vi "RFmx_Cntr_Init_Complete.vi"(7 "Meas_Type":string[](array[string])=["ACP"], 8 "error in (no error)":errorcluster, 11 "Instrument Handle in":refnum<k21>="VST") -> (0 "error out":errorcluster, 3 "Instrument Handle out":refnum<k21>="VST")   [LabVIEW 2014]
uses:
  <vilib>/RFmx/RFInstr/mx/RFmxInstr.llb/RFmxInstr Build Signal String.vi
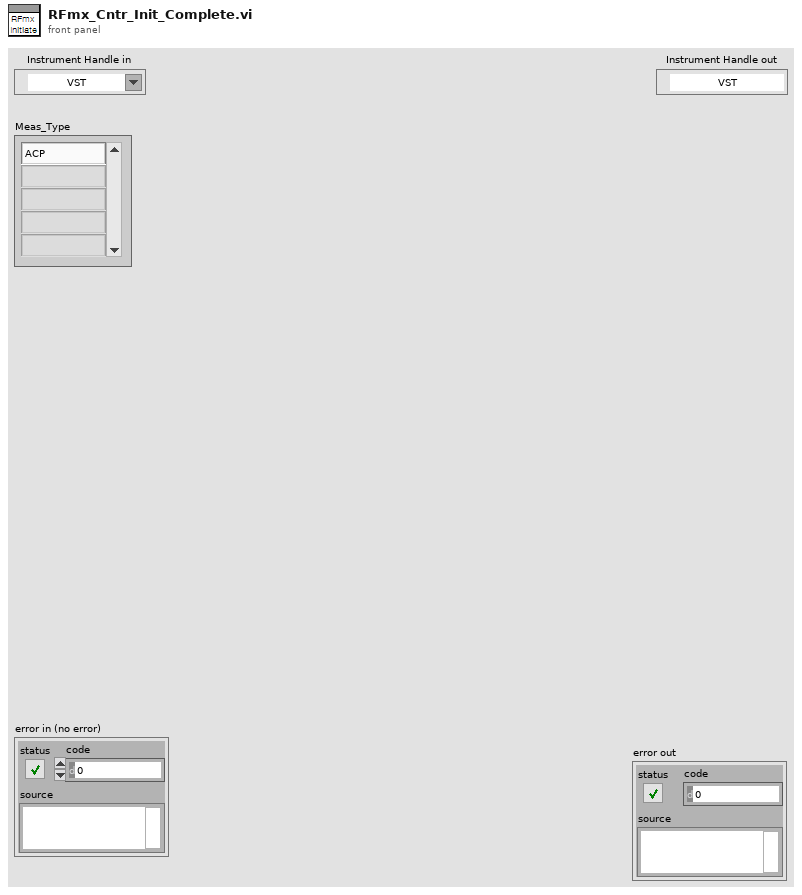
[diagram p1: front panel]
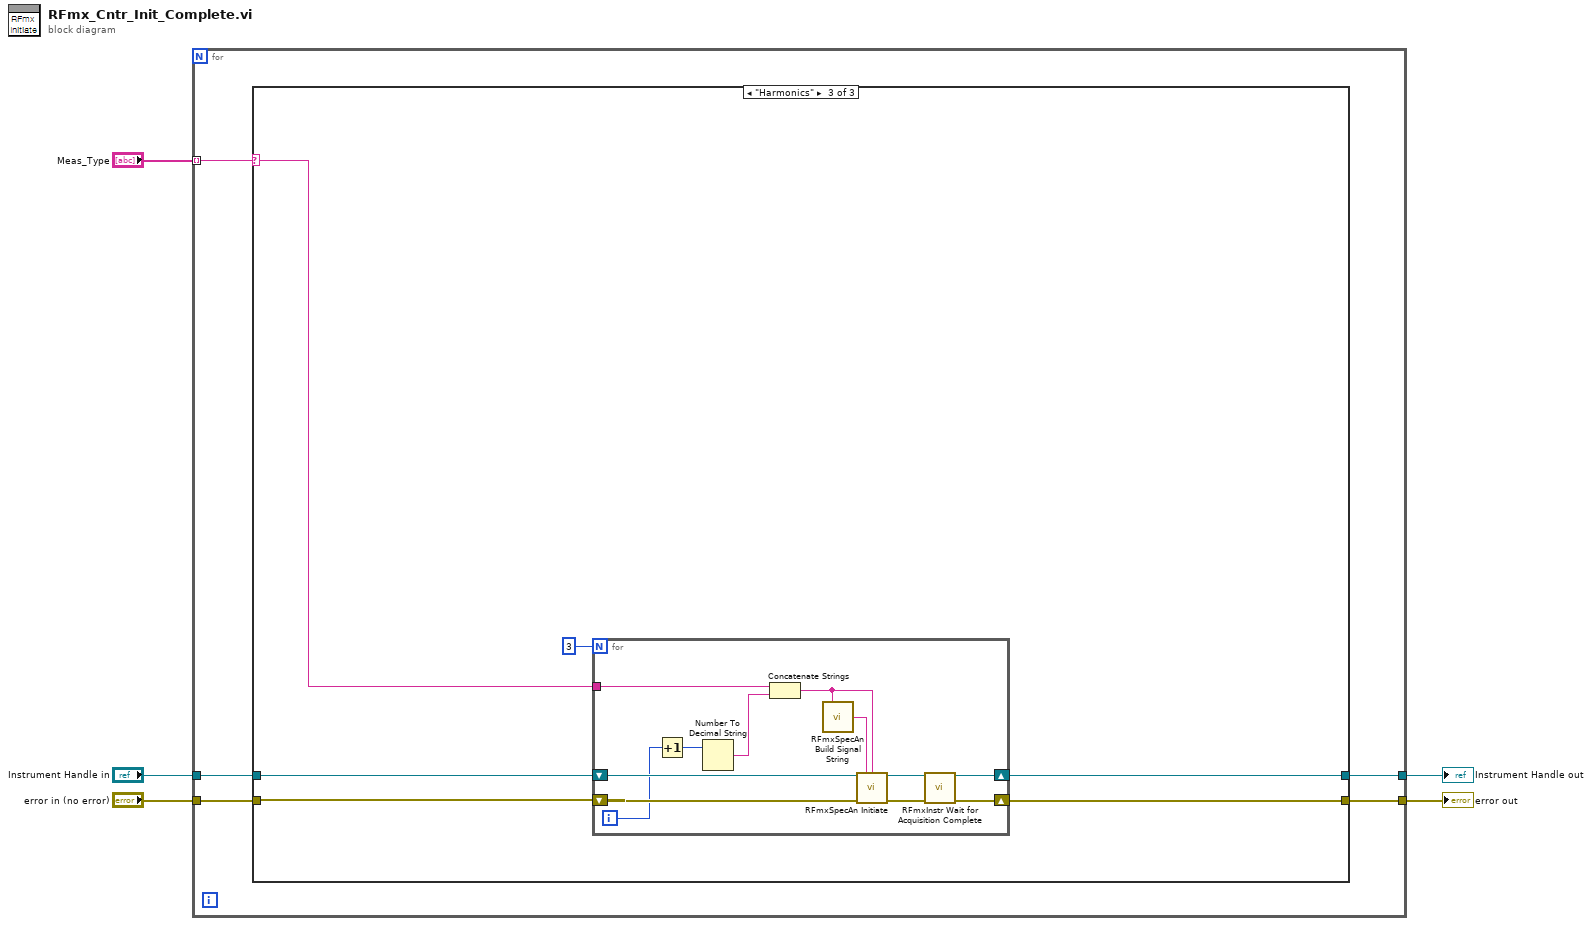
[diagram p0: block diagram]
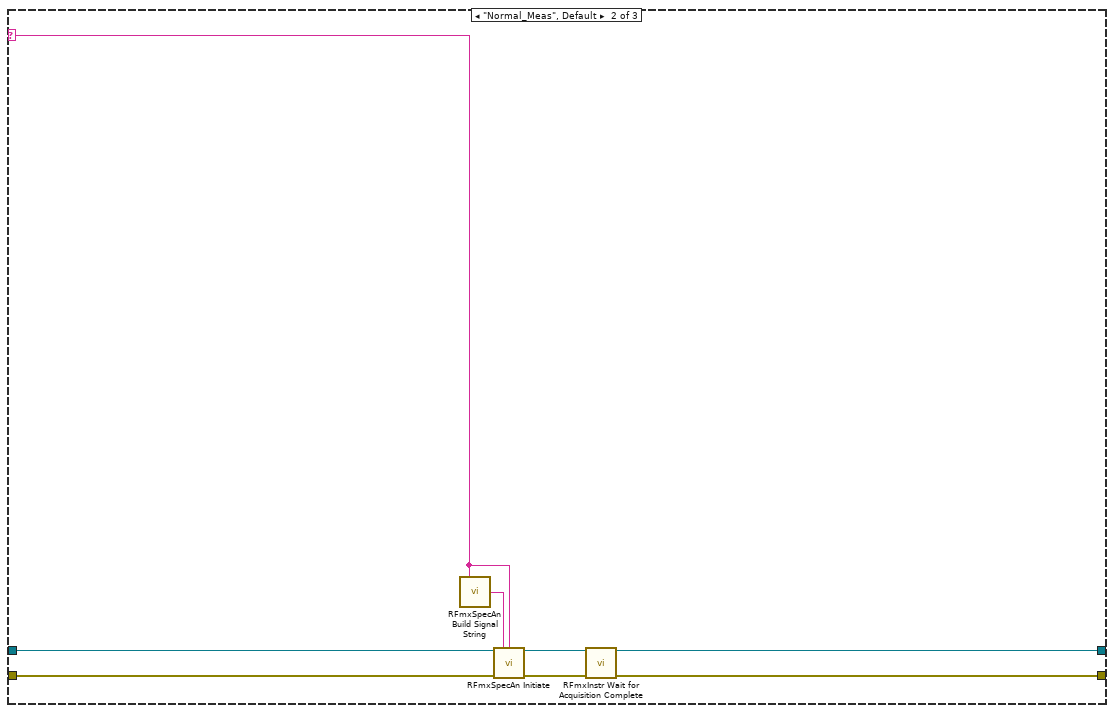
[diagram p3: hidden frame]
diagram:
  n1 = for {
    tunnel: [w10] -> w5
    tunnel: [w9] -> w4
    tunnel: "Meas_Type" -> [w8] mode=indexing
    tunnel: "Instrument Handle in" -> [w7]
    tunnel: "error in (no error)" -> [w6]
    n2 = case shown="\"Harmonics\"" w8 {
      selector: w8 -> [_ w15 w21]
      tunnel: w7 -> [w12 w17 w25]
      tunnel: w6 -> [w11 w16 w24]
      tunnel: [w12 w14 w23] -> w9
      tunnel: [w11 w13 w22] -> w10
      frame "Nothing" {
      }
      frame "Normal_Meas", Default {
        n3 = call <vilib>:"RFmxSpecAn Build Signal String.vi"("Signal Name"=w15) -> ("Selector String"=w20:string)  [unwired: 14 in]
        n4 = call <vilib>:"RFmxSpecAn Initiate.vi"("Instrument Handle In"=w17, "Selector String"=w20, "Result Name"=w15, "error in (no error)"=w16) -> ("Instrument Handle Out"=w19:refnum<k21>, "error out"=w18:errorcluster)  [unwired: 9 in, 1 out]
        n5 = call <vilib>:"RFmxInstr Wait for Acquisition Complete.vi"("Instrument Handle In"=w19, "error in (no error)"=w18) -> ("Instrument Handle Out"=w14:refnum<k21>, "error out"=w13:errorcluster)  [unwired: 12 in]
      }
      frame "Harmonics" {
        n6 = for {
          N: 3 -> [_]
          shift-right: [w32] -> w23
          shift-left: w25 -> [w38]
          shift-right: [w33] -> w22
          shift-left: w24 -> [w37]
          tunnel: w21 -> [w27]
          i -> [w29]
          n7 = Increment(x=w29) -> (x+1=w28:i32)
          n8 = Number To Decimal String(number=w28) -> (decimal integer string=w31:string)  [unwired: 1 in]
          n9 = Concatenate Strings(w27, w31) -> (w30:string)
          n10 = call <vilib>:"RFmxSpecAn Build Signal String.vi"("Signal Name"=w30) -> ("Selector String"=w36:string)  [unwired: 14 in]
          n11 = call <vilib>:"RFmxSpecAn Initiate.vi"("Instrument Handle In"=w38, "Selector String"=w36, "Result Name"=w30, "error in (no error)"=w37) -> ("Instrument Handle Out"=w35:refnum<k21>, "error out"=w34:errorcluster)  [unwired: 9 in, 1 out]
          n12 = call <vilib>:"RFmxInstr Wait for Acquisition Complete.vi"("Instrument Handle In"=w35, "error in (no error)"=w34) -> ("Instrument Handle Out"=w32:refnum<k21>, "error out"=w33:errorcluster)  [unwired: 12 in]
        }
      }
    }
  }
  "Instrument Handle out" <- w4
  "error out" <- w5
